vi "set_boost_type.vi"(6 "timeout (25000ms)":i32=25000, 8 "error in (no error)":errorcluster, 10 "Boost type":T1, 11 "daemon reference in":refnum<k5>) -> (0 "error out":errorcluster, 2 "response":string, 3 "daemon reference out":refnum<k5>, 5 "command out":string="random")   [LabVIEW 2017]
doc: "<b>Command: </b>\"set_boost_type\"\n\n<b>Description: </b> This command set boost type.\n\n<b>Parameters: </b> boost type\n____________________________________________\nDIPC 692 Daemon API 10.0.0.1\nSam Tee - Dyson Technology Ltd\nCopyright (c) 2024, Dyson Technology Ltd"
uses:
  typdef/boost_type.ctl
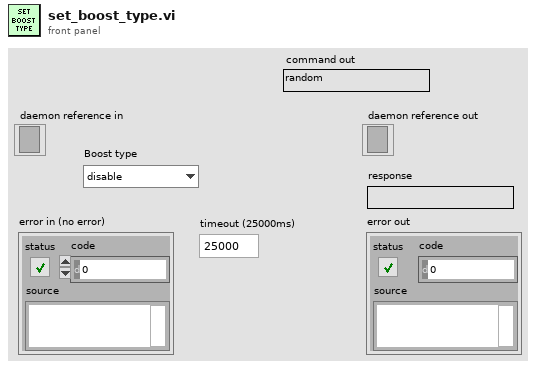
[diagram p1: front panel]
types:
  T1 = typedef "boost_type.ctl" = enum16{"disable", "normal", "high"}
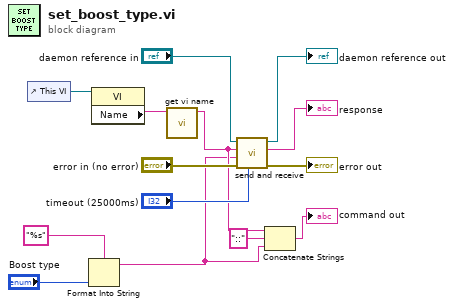
[diagram p0: block diagram]
diagram:
  n1 = control-ref of="This VI"() -> (w8:refnum<vi>)
  n2 = Format Into String(format string="%s" ("initial string"), "Boost type") -> (resulting string=w1:string)  [unwired: 2 in, 1 out]
  n3 = property class="VI"(reference=w8) -> ("Name"=w7:string)  [unwired: 1 in, 2 out]
  n4 = call "get vi name.vi"("library.lvlib:name.vi"=w7) -> ("vi name"=w3:string)  [unwired: 10 in]
  n5 = call "send and receive.vi"("timeout (25000ms)"="timeout (25000ms)", "error in (no error)"="error in (no error)", "data"=w1, "command"=w3, "daemon reference in"="daemon reference in") -> ("error out"=→"error out":errorcluster, "response"=→"response":string, "daemon reference out"=→"daemon reference out":refnum<k5>)  [unwired: 4 in]
  n6 = Concatenate Strings(w3, "::" ("string"), w1) -> (→"command out":string)
